vi "Launch Data Type Config.vi"(8 "error in (no error)":errorcluster, 10 "Selection":i32, 11 "DataGrid Config Dialog in":refnum<class "DataGrid Config Dialog.lvclass">) -> (0 "error out":errorcluster, 3 "DataGrid Config Dialog out":refnum<class "DataGrid Config Dialog.lvclass">)   [LabVIEW 2018, in "DataGrid Config Dialog.lvclass"]
uses:
  DataGrid Config Dialog.lvclass
  DataGrid Config Dialog.lvclass/DataGrid Config Dialog.ctl
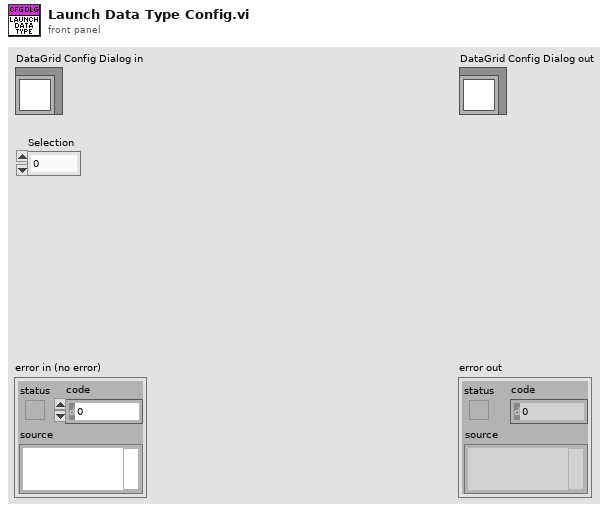
[diagram p1: front panel]
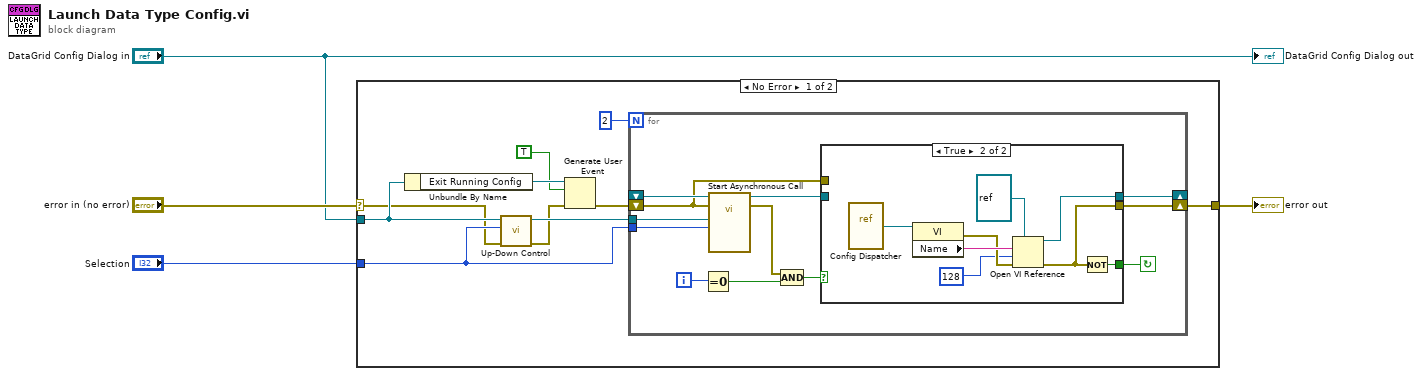
[diagram p0: block diagram]
diagram:
  n1 = case shown="No Error" "error in (no error)" {
    selector: "error in (no error)" -> [w6 w37]
    tunnel: "DataGrid Config Dialog in" -> [w9 _]
    tunnel: [w13 w37] -> w3
    tunnel: "Selection" -> [w7 _]
    frame No Error {
      n2 = Unbundle By Name(w9) -> ("Exit Running Config"=w12:refnum<user-event>)
      n3 = call "Up-Down Control.vi"("error in (no error)"=w6, "Selection"=w7, "DataGrid Config Dialog in"=w9) -> ("error out"=w5:errorcluster, "DataGrid Config Dialog out"=w8:refnum<class "DataGrid Config Dialog.lvclass">)  [unwired: 7 in]
      n4 = Generate User Event(user event=w12, event data cluster=TRUE, error in=w5) -> (error out=w11:errorcluster)  [unwired: 1 in, 1 out]
      n5 = for {
        N: 2 -> [_]
        tunnel: w8 -> [w26]
        shift-right: [w23] -> _
        shift-left: _ -> [w25]
        shift-right: [w17] -> w13
        shift-left: w11 -> [w16]
        tunnel: w7 -> [w15]
        i -> [w21]
        stop <- w22 continue-if-true
        n6 = Equal To 0?(x=w21) -> (x = 0?=w20:bool)
        n7 = call-by-ref "Start Asynchronous Call"(reference=w25, error in=w16, "Selection"=w15, "DataGrid Config Dialog in"=w26) -> (reference out=w24:refnum<vi>, error out=w19:errorcluster)  [unwired: 8 in, 2 out]
        n8 = Compound Arithmetic op=AND(w19, w20) -> (w18:bool)
        n9 = case shown="True" w18 {
          tunnel: w24 -> [w28 _]
          tunnel: [w28 w31] -> w23
          tunnel: [_ w30] -> w22
          tunnel: [w27 w29] -> w17
          tunnel: w16 -> [w27 _]
          frame False {
          }
          frame True {
            n10 = vi-ref "Config Dispatcher.vi"() -> (w36:refnum<vi>)
            n11 = property class="VI"(reference=w36) -> (error out=w34:errorcluster, "Name"=w35:string)  [unwired: 1 in, 1 out]
            n12 = Open VI Reference(type specifier VI Refnum (for type only)=refnum<vi> refnum, vi path=w35, options=128, error in (no error)=w34) -> (vi reference=w31:refnum<vi>, error out=w29:errorcluster)  [unwired: 2 in]
            n13 = Not(x=w29) -> (.not. x?=w30:bool)
          }
        }
      }
    }
    frame Error {
    }
  }
  "error out" <- w3
  "DataGrid Config Dialog out" <- "DataGrid Config Dialog in"
